vi "DB Tools Format Datetime String.vi"   [LabVIEW 2012, in "NI_Database_API_64.lvlib"]
doc: "Returns a string containing the formatted date and time, and identifies the string as a date/time string so other VIs can interpret this string. Wire data to the input of this VI to determine the polymorphic instance to use or manually select the instance."
uses:
  NI_Database_API_64.lvlib
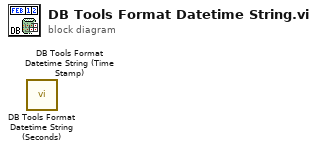
[diagram p0: block diagram]
diagram:
  n1 = call "DB Tools Format Datetime String (Seconds).vi"() -> ()  [unwired: 1 in, 1 out]
  n2 = call "DB Tools Format Datetime String (Time Stamp).vi"() -> ()  [unwired: 1 in, 1 out]
